vi "Generate Temporary Report.vi"(8 "error in (no error)":errorcluster, 10 "Line of Events":string[](array[string]), 11 "Module Name":string) -> (0 "error out":errorcluster)   [LabVIEW 2018, in "Report Generation.lvlib"]
uses:
  Report Generation.lvlib
  <vilib>/Utility/file.llb/Write Delimited Spreadsheet (string).vi
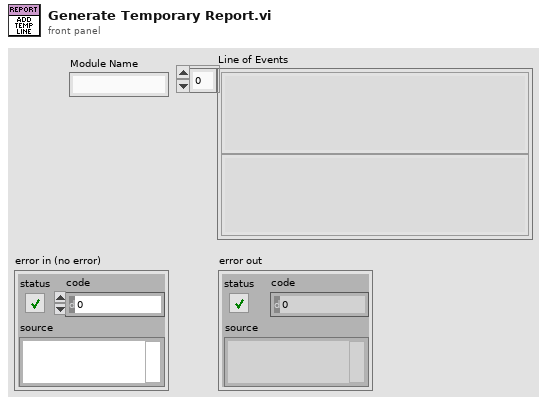
[diagram p1: front panel]
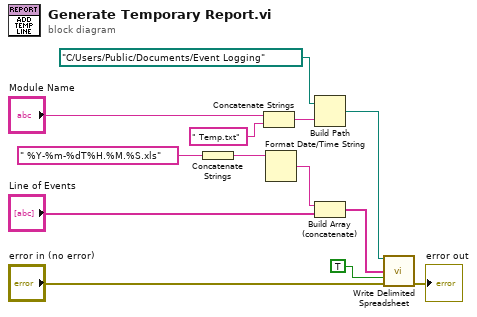
[diagram p0: block diagram]
diagram:
  n1 = Concatenate Strings(" %Y-%m-%dT%H.%M.%S.xls" ("time format string (%c)")) -> (w2:string)
  n2 = Concatenate Strings("Module Name", " Temp.txt" ("string")) -> (w8:string)
  n3 = Format Date/Time String(time format string (%c)=w2) -> (date/time string=w1:string)  [unwired: 2 in]
  n4 = Build Path(base path=path "C:/Users/Public/Documents/Event Logging" ("file path (dialog if empty)"), name or relative path=w8) -> (appended path=w10:path)
  n5 = Build Array (concatenate)(w1, "Line of Events") -> (w4:string[])
  n6 = call-poly <vilib>:"Write Delimited Spreadsheet.vi"("file path (dialog if empty)"=w10, "1D data"=w4, "append to file? (new file:F)"=TRUE, "error in (no error)"="error in (no error)") -> ("error out"=→"error out":errorcluster)  [unwired: 10 in, 1 out]
